vi "Decimate image v2.vi"(9 "Image Pixels (U8)":sgl[][](array[numeric]), 10 "Target array":sgl[][](array[numeric]), 11 "Decimate by N":i32) -> (3 "Filled target array":sgl[][](array[numeric]))   [LabVIEW 2018]
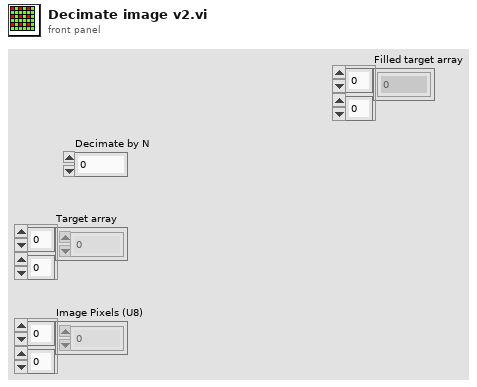
[diagram p1: front panel]
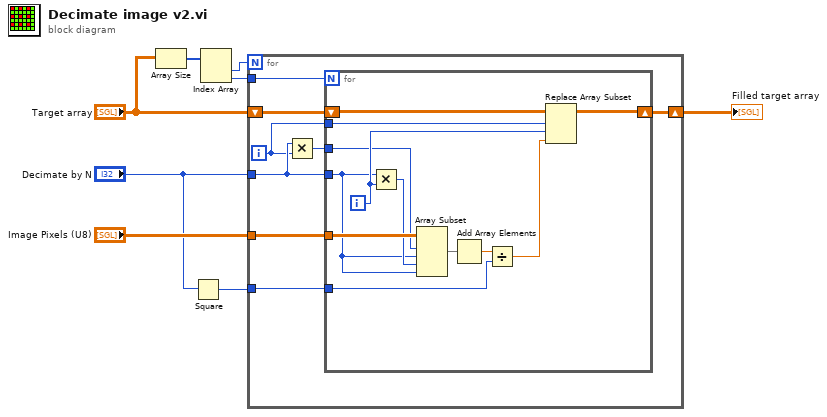
[diagram p0: block diagram]
diagram:
  n1 = Array Size(array="Target array") -> (size(s)=w8:i32[])
  n2 = Square(x="Decimate by N") -> (x^2=w1:i32)
  n3 = Index Array(array=w8) -> (element #1=w7:i32, element #2=w6:i32)  [unwired: 2 in]
  n4 = for {
    N: w7 -> [_]
    tunnel: w6 -> [w16]
    tunnel: "Decimate by N" -> [w13]
    shift-right: [w11] -> w3
    shift-left: "Target array" -> [w15]
    tunnel: "Image Pixels (U8)" -> [w10]
    tunnel: w1 -> [w9]
    i -> [w12]
    n5 = Multiply(x=w13, y=w12) -> (x*y=w14:i32)
    n6 = for {
      N: w16 -> [_]
      tunnel: w14 -> [w23]
      tunnel: w13 -> [w20]
      tunnel: w12 -> [w27]
      shift-right: [w25] -> w11
      shift-left: w15 -> [w28]
      tunnel: w10 -> [w24]
      tunnel: w9 -> [w17]
      i -> [w26]
      n7 = Multiply(x=w20, y=w26) -> (x*y=w21:i32)
      n8 = Array Subset(array=w24, index (row)=w23, length (row)=w20, index (col)=w21, length (col)=w20) -> (w22:sgl[][])
      n9 = Add Array Elements(numeric array=w22) -> (sum=w19:sgl)
      n10 = Divide(x=w19, y=w17) -> (x/y=w18:sgl)
      n11 = Replace Array Subset(array=w28, new element=w18, index (row)=w27, index (col)=w26) -> (w25:sgl[][])
    }
  }
  "Filled target array" <- w3
